vi "氨氮测量数据储存.vi"   [LabVIEW 2016, in "斯坦道氨氮.lvlib"]
types:
  T1 = cluster{"时间标识":timestamp, "监测值":sgl, "单位":u16, "数据标识":string, "因子编码":u32, "标样参考值":sgl, "F0":sgl, "F1":sgl, "F2":sgl, "F3":sgl, "F4":sgl, "F5":sgl, "F6":sgl, "F7":sgl, "T":sgl, "H":sgl, "X":sgl, "量程标识":string}
  T2 = enum16{"维护数据", "水样测试", "标样核查", "零点核查", "跨度核查", "空白测试", "平行样测试", "加标回收", "空白校准", "标样校准", "初始化（清洗）"}
  T3 = cluster{"系统时间":timestamp, "工作状态":enum16{"空闲", "水样测试", "标样核查", "零点核查", "跨度核查", "空白测试", "平行样测试", "加标回收", "空白校准", "标样校准", "初始化（清洗）"}, "测量模式":enum16{"待机", "连续模式", "周期模式", "定点模式", "受控模式", "手动模式"}, "告警代码":enum16{"无告警", "缺试剂告警", "缺水样告警", "缺蒸馏水告警", "缺标液告警", "仪表漏液告警", "标定异常告警", "超量程告警", "加热异常", "低试剂预警", "超上限告警", "超下限告警", "仪表内部其他异常", "滴定异常告警", "电极异常告警", "量程切换告警", "参数设置告警", "PH电极电位异常", "电导率电极异常", "浊度光度异常", "溶解氧电极异常", "溶解氧光强异常", "温度异常告警", "PH异常告警", "溶解氧异常告警", "电导率异常告警", "浊度异常告警", "叶绿素异常告警", "藻密度异常告警", "蓝绿藻异常告警", "ORP异常告警", "氨氮异常告警", "清洁刷异常告警", "SD卡异常告警", "蓝牙异常告警", "Wifi异常告警", "流程异常告警"}, "故障代码":enum16{"无故障", "电机故障", "温度故障", "通讯故障", "滴定故障"}, "日志代码":u16, "软件版本":u16, "F0":sgl, "F1":sgl, "F2":sgl, "F3":sgl, "T":sgl, "H":sgl, "id":u16, "flowid":u16, "量程":u16, "总磷控温温度1":sgl, "营养盐控温温度2":sgl, "ADC":sgl}
  T4 = enum16{"空闲", "水样测试", "标样核查", "零点核查", "跨度核查", "空白测试", "平行样测试", "加标回收", "空白校准", "标样校准", "初始化（清洗）"}
  T5 = cluster{"运行模式":enum16{"维护模式", "常规模式", "应急模式", "质控模式"}, "质控频次":enum16{"关闭", "每天", "星期一", "星期二", "星期三", "星期四", "星期五", "星期六", "星期日"}, "空白核查时间":u16, "跨度核查时间":u16, "24H周期设置":bool[]}
  T6 = cluster{"跨度值":dbl, "零点标准液浓度":dbl, "跨度标准液浓度":dbl, "标准液标准浓度":dbl}
  T7 = cluster{"因子编码":u32, "单位":u16, "标样参考值":sgl, "水样数据时间":timestamp, "水样实测值":sgl, "水样数据标识":string, "标样数据时间":timestamp, "标样实测值":sgl, "标样数据标识":string, "空白数据时间":timestamp, "空白实测值":sgl, "空白数据标识":string, "零点核查数据时间":timestamp, "零点核查实测值":sgl, "零点核查数据标识":string, "跨度核查数据时间":timestamp, "跨度核查实测值":sgl, "跨度核查数据标识":string, "加标回收数据时间":timestamp, "加标回收实测值":sgl, "加标回收数据标识":string, "平行样数据时间":timestamp, "平行样实测值":sgl, "平行样数据标识":string, "F0":sgl, "F1":sgl, "F2":sgl, "F3":sgl, "F4":sgl, "F5":sgl, "F6":sgl, "F7":sgl, "T":sgl, "H":sgl, "X":sgl}
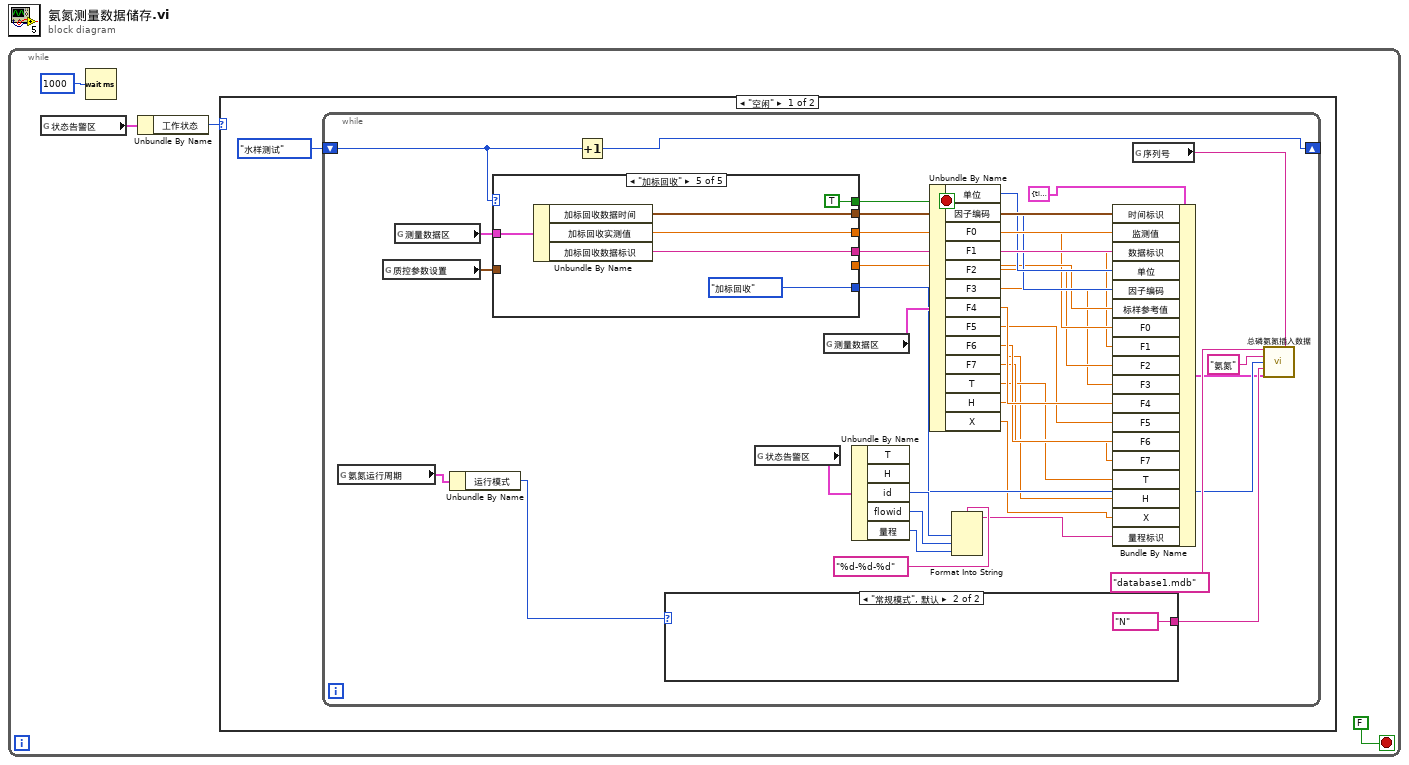
[diagram p0: block diagram]
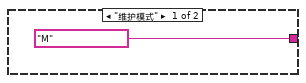
[diagram p2: hidden frame]
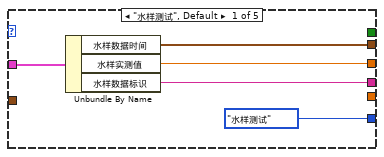
[diagram p3: hidden frame]
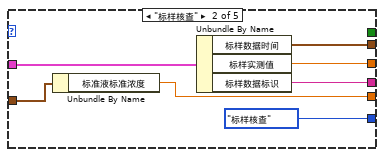
[diagram p4: hidden frame]
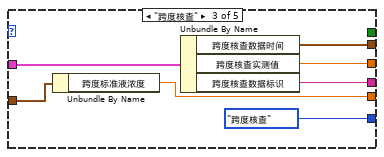
[diagram p5: hidden frame]
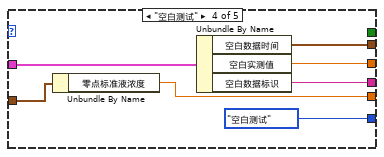
[diagram p6: hidden frame]
diagram:
  n1 = while {
    stop <- FALSE stop-if-true
    n2 = global read "VAR氨氮全局变量.vi" "状态告警区"() -> (w3:T3)
    n3 = Wait (ms)(milliseconds to wait=u32 1000 ("等待时间（毫秒）")) -> ()  [unwired: 1 out]
    n4 = Unbundle By Name(w3) -> ("工作状态"=w2:T4)
    n5 = case shown="\"空闲\"" w2 {
      frame "空闲" {
        n6 = while {
          shift-right: [w37] -> _
          shift-left: enum16{"水样测试", "标样核查", "跨度核查", "空白测试", "加标回收"}."水样测试" ("测量模式") -> [w38]
          stop <- w39 stop-if-true
          n7 = global read "氨氮断电保存全局变量.vi" "氨氮运行周期"() -> (w20:T5)
          n8 = global read "氨氮断电保存全局变量.vi" "质控参数设置"() -> (w22:T6)
          n9 = global read "VAR氨氮全局变量.vi" "测量数据区"() -> (w31:T7)
          n10 = Unbundle By Name(w20) -> ("运行模式"=w19:enum16{"维护模式", "常规模式", "应急模式", "质控模式"})
          n11 = case shown="\"加标回收\"" w38 {
            tunnel: w31 -> [w46 w53 w60 w67 w72]
            tunnel: [w50 w57 w64 w71 w77] -> w36
            tunnel: [w49 w56 w63 w70 w76] -> w35
            tunnel: [w48 w55 w62 w69 w75] -> w34
            tunnel: [T2."水样测试" ("测量模式") T2."标样核查" ("测量模式") T2."跨度核查" ("测量模式") T2."空白测试" ("测量模式") T2."加标回收" ("测量模式")] -> w25
            tunnel: [_ _ _ _ TRUE] -> w39
            tunnel: w22 -> [_ w52 w59 w66 _]
            tunnel: [_ w51 w58 w65 _] -> w21
            frame "水样测试", Default {
              n12 = Unbundle By Name(w46) -> ("水样数据时间"=w50:timestamp, "水样实测值"=w49:sgl, "水样数据标识"=w48:string)
            }
            frame "标样核查" {
              n13 = Unbundle By Name(w52) -> ("标准液标准浓度"=w51:dbl)
              n14 = Unbundle By Name(w53) -> ("标样数据时间"=w57:timestamp, "标样实测值"=w56:sgl, "标样数据标识"=w55:string)
            }
            frame "跨度核查" {
              n15 = Unbundle By Name(w59) -> ("跨度标准液浓度"=w58:dbl)
              n16 = Unbundle By Name(w60) -> ("跨度核查数据时间"=w64:timestamp, "跨度核查实测值"=w63:sgl, "跨度核查数据标识"=w62:string)
            }
            frame "空白测试" {
              n17 = Unbundle By Name(w66) -> ("零点标准液浓度"=w65:dbl)
              n18 = Unbundle By Name(w67) -> ("空白数据时间"=w71:timestamp, "空白实测值"=w70:sgl, "空白数据标识"=w69:string)
            }
            frame "加标回收" {
              n19 = Unbundle By Name(w72) -> ("加标回收数据时间"=w77:timestamp, "加标回收实测值"=w76:sgl, "加标回收数据标识"=w75:string)
            }
          }
          n20 = Increment(x=w38) -> (x+1=w37:enum16{"水样测试", "标样核查", "跨度核查", "空白测试", "加标回收"})
          n21 = case shown="\"常规模式\", 默认" w19 {
            tunnel: ["M" ("数据标记表") "N" ("数据标记表")] -> w23
            frame "维护模式" {
            }
            frame "常规模式", Default {
            }
          }
          n22 = global read "VAR氨氮全局变量.vi" "状态告警区"() -> (w29:T3)
          n23 = global read "VAR氨氮全局变量.vi" "测量数据区"() -> (w30:T7)
          n24 = Unbundle By Name(w29) -> ("id"=w42:u16, "flowid"=w41:u16, "量程"=w40:u16)  [unwired: 2 out]
          n25 = Unbundle By Name(w30) -> ("单位"=w33:u16, "因子编码"=w32:u32, "F0"=w18:sgl, "F1"=w17:sgl, "F2"=w16:sgl, "F3"=w15:sgl, "F4"=w12:sgl, "F5"=w11:sgl, "F6"=w10:sgl, "F7"=w9:sgl, "T"=w8:sgl, "H"=w7:sgl, "X"=w6:sgl)
          n26 = Format Into String(format string="%d-%d-%d" ("格式字符串"), w42, w41, w40) -> (resulting string=w24:string)  [unwired: 2 in, 1 out]
          n27 = Bundle By Name(cluster=T1 {"时间标识"=timestamp(0 s since 1904-01-01), "监测值"=0.0, "单位"=0, "数据标识"="", "因子编码"=0, "标样参考值"=0.0, "F0"=0.0, "F1"=0.0, "F2"=0.0, "F3"=0.0, "F4"=0.0, "F5"=0.0, "F6"=0.0, "F7"=0.0, "T"=0.0, "H"=0.0, "X"=0.0, "量程标识"=""} ("data"), "时间标识"=w36, "监测值"=w35, "数据标识"=w34, "单位"=w33, "因子编码"=w32, "标样参考值"=w21, "F0"=w18, "F1"=w17, "F2"=w16, "F3"=w15, "F4"=w12, "F5"=w11, "F6"=w10, "F7"=w9, "T"=w8, "H"=w7, "X"=w6, "量程标识"=w24) -> (w13:T1)
          n28 = global read "VAR氨氮全局变量.vi" "序列号"() -> (w28:string)
          n29 = call "总磷氨氮插入数据.vi"("database"="database1.mdb", "data"=w13, "SN"=w28, "table"="氨氮", "测量模式"=w25, "数据标记表"=w23) -> ()  [unwired: 9 in, 1 out]
        }
      }
      frame "水样测试", Default {
      }
    }
  }
